vi "Wait.vi"() -> ()   [LabVIEW 2015]
panel:
  in  "milliseconds to wait array":u32[](array[numeric])=[500, 500, 500, 500, 500, 500, 500, 500]
  # "PROCESSES"
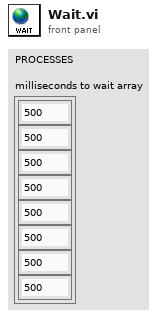
[diagram p1: front panel]
diagram:
